vi "Load layout to marking engine.vi"(8 "error in (no error)":errorcluster, 10 "layout to load":string, 11 "Domino Laser module Class in":refnum<class "Domino Laser module Class.lvclass">) -> (0 "error out":errorcluster, 3 "Domino Laser module Class out":refnum<class "Domino Laser module Class.lvclass">)   [LabVIEW 2015, in "Domino LM.lvlib" / "Domino Laser module Class.lvclass"]
uses:
  CTRLS/Domino Laser module Class.lvclass
  CTRLS/Domino Laser module Class.lvclass/Domino Laser module Class.ctl
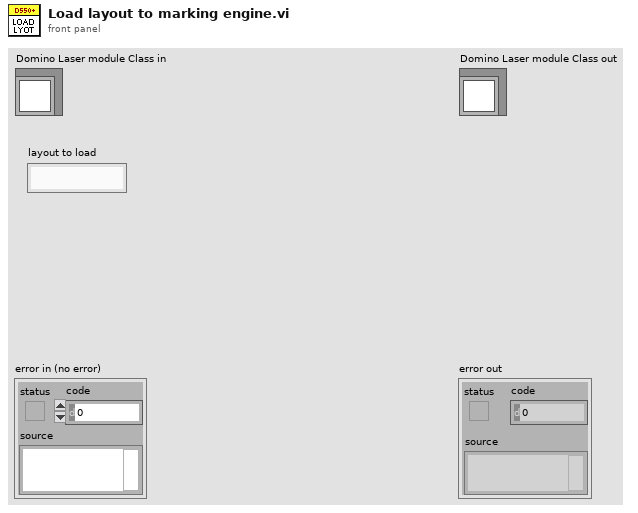
[diagram p1: front panel]
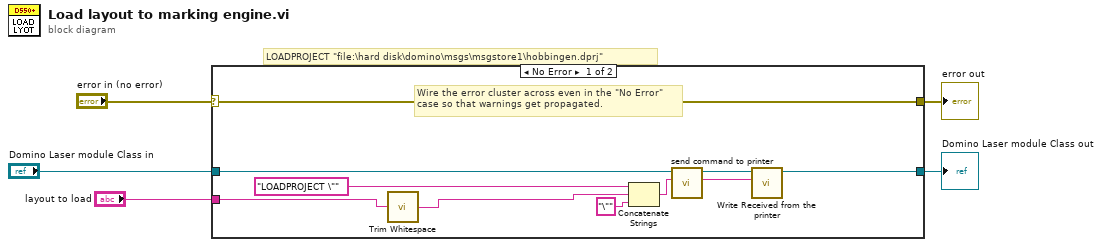
[diagram p0: block diagram]
diagram:
  # "LOADPROJECT \"file:\\hard disk\\domino\\msgs\\msgstore1\\hobbingen.dprj\""
  n1 = case shown="No Error" "error in (no error)" {
    selector: "error in (no error)" -> [w15 w17]
    tunnel: [w15 w17] -> w4
    tunnel: [w9 w16] -> w2
    tunnel: "Domino Laser module Class in" -> [w14 w16]
    tunnel: "layout to load" -> [w7 _]
    frame No Error {
      # "Wire the error cluster across even in the \"No Error\"\ncase so that warnings get propagated."
      n2 = call <vilib>:"Trim Whitespace.vi"("string"=w7) -> ("trimmed string"=w6:string)  [unwired: 1 in]
      n3 = Concatenate Strings("LOADPROJECT \"", w6, "\"" ("string")) -> (w11:string)
      n4 = call "send command to printer.vi"("command to be sent"=w11, "Domino Laser module Class in"=w14) -> ("Recived message"=w8:string, "Domino Laser module Class out"=w10:refnum<class "Domino Laser module Class.lvclass">)  [unwired: 6 in, 2 out]
      n5 = call "Write Received from the printer.vi"("Received from the printer"=w8, "Domino Laser module Class in"=w10) -> ("Domino Laser module Class out"=w9:refnum<class "Domino Laser module Class.lvclass">)  [unwired: 8 in, 1 out]
    }
    frame Error {
    }
  }
  "error out" <- w4
  "Domino Laser module Class out" <- w2
